vi "sub_pf_motion-model.vi"(10 "u":T1, 11 "x_true":T1) -> (3 "x_true out":T1)   [LabVIEW 2019]
uses:
  <vilib>/Analysis/Matrix/Datatypes/RealMatrix.ctl
  Ctrl/cmd_common.ctl
  <vilib>/Analysis/Matrix/Numeric/Multiply/Multiply - RM,RM.vi
  <vilib>/Analysis/Matrix/Numeric/Add/Add - RM,RM.vi
  <vilib>/Analysis/Matrix/NI_Matrix.lvlib
panel:
  out "행 x_true":i32
  out "열 x_true":i32
  out "열 F":i32
  out "행 F":i32
  out "B":T1
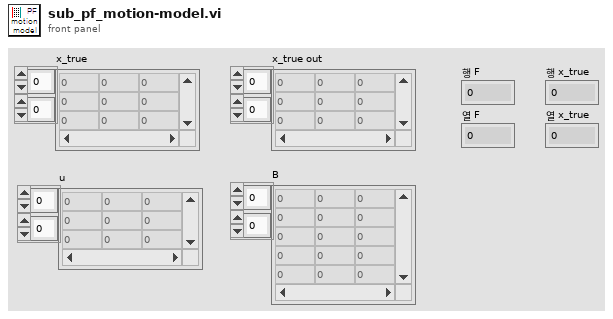
[diagram p1: front panel]
types:
  T1 = typedef "NI_Matrix.lvlib/RealMatrix.ctl" = dbl[][]
  T2 = typedef "cmd_common.ctl" = enum16{"read", "write"}
  T3 = cluster{"DT":dbl, "SIM_TIME":dbl, "MAX_RANGE":dbl, "NP":u32, "NTh":u32, "Q":T1, "R":T1, "Q_sim":T1, "R_sim":T1, "rf_id":cluster{"x":dbl, "y":dbl}[]}
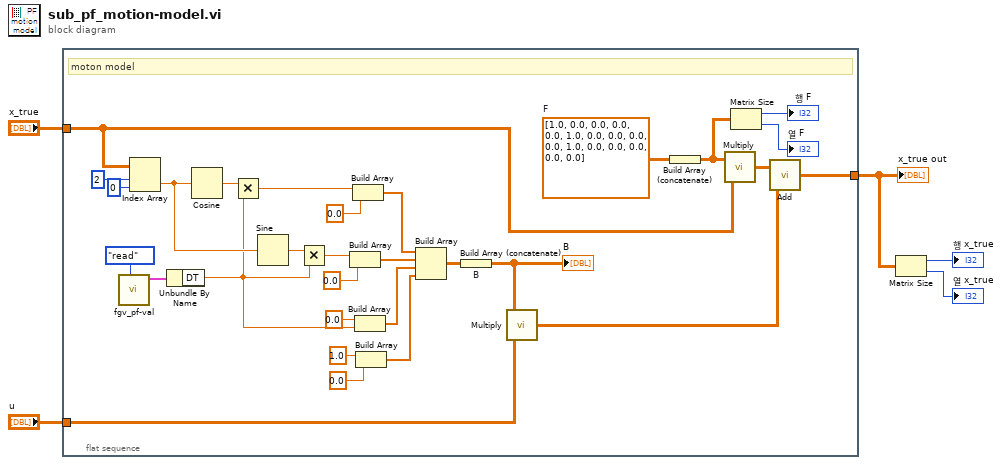
[diagram p0: block diagram]
diagram:
  n1 = flat-sequence {
    tunnel: "x_true" -> [w15]
    tunnel: "u" -> [w13]
    tunnel: [w9] -> w1
    frame #0 {
      w16 = dbl[][] [[1.0, 0.0, 0.0, 0.0], [0.0, 1.0, 0.0, 0.0], [0.0, 0.0, 1.0, 0.0], [0.0, 0.0, 0.0, 0.0]]  # F
      # "moton model"
      n2 = call "fgv_pf-val.vi"("cmd"=cmd_common."read") -> ("pf-val out"=w11:T3)  [unwired: 10 in]
      n3 = Index Array(array=w15, index (row)=2 ("인덱스 (행)"), index (col)=0 ("인덱스 (열)")) -> (element=w31:dbl)
      n4 = Unbundle By Name(w11) -> ("DT"=w10:dbl)
      n5 = Cosine(x=w31) -> (cos(x)=w33:dbl)
      n6 = Multiply(x=w33, y=w10) -> (x*y=w30:dbl)
      n7 = Sine(x=w31) -> (sin(x)=w32:dbl)
      n8 = Multiply(x=w32, y=w10) -> (x*y=w27:dbl)
      n9 = Build Array(w27, 0.0 ("원소")) -> (w21:dbl[])
      n10 = Build Array(w30, 0.0 ("원소")) -> (w20:dbl[])
      n11 = Build Array(0.0 ("원소"), w10) -> (w22:dbl[])
      n12 = Build Array(1.0 ("원소"), 0.0 ("원소")) -> (w23:dbl[])
      n13 = Build Array(w20, w21, w22, w23) -> (w19:dbl[][])
      n14 = Build Array (concatenate) "B"(w19) -> (w18:T1)
      "B" <- w18
      n15 = call-poly <vilib>:"Multiply.vi"("Real Matrix B"=w13, "Real Matrix A"=w18) -> ("A * B"=w17:T1)
      n16 = Build Array (concatenate)(w16) -> (w8:T1)
      n17 = call-poly <vilib>:"Multiply.vi"("Real Matrix B"=w15, "Real Matrix A"=w8) -> ("A * B"=w14:T1)
      n18 = Matrix Size(0:w8) -> (1:→"행 F":i32, 2:→"열 F":i32)
      n19 = call-poly <vilib>:"Add.vi"("Real Matrix B"=w17, "Real Matrix A"=w14) -> ("A + B"=w9:T1)
    }
  }
  n20 = Matrix Size(0:w1) -> (1:→"행 x_true":i32, 2:→"열 x_true":i32)
  "x_true out" <- w1
